vi "SimpleExportUseBookmark.vi"(4 "GraphBookmark":string, 5 "StringData":string[](array[string]), 6 "GraphReference":refnum<vi>, 7 "BookmarkTarget":string[](array[string]), 8 "error in (no error)":errorcluster, 10 "TemplateFilePath":path) -> (0 "error out":errorcluster)   [LabVIEW 2013]
uses:
  <vilib>/Utility/NIReport.llb/NI_report.lvclass
  <vilib>/Utility/NIReport.llb/Append Report Text (str wrap).vi
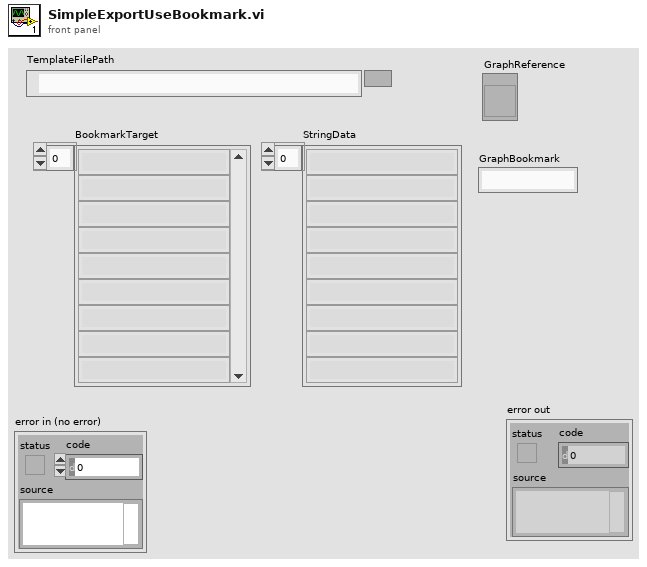
[diagram p1: front panel]
types:
  T1 = cluster{"position (excel)":cluster{"row":i32, "column":i32}, "name (excel)":string, "bookmark (word)":string}
  T2 = enum16{"Standard Report", "HTML", "Word", "Excel"}
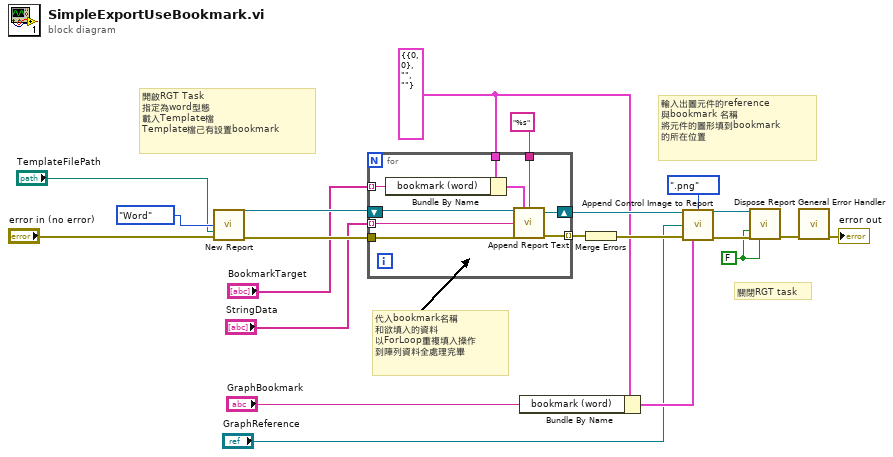
[diagram p0: block diagram]
diagram:
  w5 = FALSE ("save changes? (F)")
  w10 = T1 {"position (excel)"={"row"=0, "column"=0}, "name (excel)"="", "bookmark (word)"=""} ("MS Office parameters")
  # "關閉RGT task"
  # "輸入出圖元件的reference\n與bookmark 名稱\n將元件的圖形填到bookmark\n的所在位置"
  # "代入bookmark名稱\n和欲填入的資料\n以ForLoop重複填入操作\n到陣列資料全處理完畢"
  # "開啟RGT Task\n指定為word型態\n載入Template檔\nTemplate檔己有設置bookmark"
  n1 = call <vilib>:"New Report.vi"("report type"=T2."Word", "template (empty)"="TemplateFilePath", "error in (no error)"="error in (no error)") -> ("report out"=w19:refnum<class "NI_report.lvclass">, "error out"=w18:errorcluster)  [unwired: 11 in]
  n2 = for {
    tunnel: w10 -> [w30]
    tunnel: w18 -> [w27]
    tunnel: "BookmarkTarget" -> [w26] mode=indexing
    tunnel: "StringData" -> [w25] mode=indexing
    tunnel: "%s" ("format string (%.3f)") -> [w24]
    shift-right: [w23] -> w14
    shift-left: w19 -> [w28]
    tunnel: [w22] -> w13 mode=indexing
    n3 = Bundle By Name(cluster=w30, "bookmark (word)"=w26) -> (w29:T1)
    n4 = call-poly <vilib>:"Append Report Text.vi"("report in"=w28, "MS Office parameters"=w29, "format string (%.3f)"=w24, "text"=w25, "error in (no error)"=w27) -> ("report out"=w23:refnum<class "NI_report.lvclass">, "error out"=w22:errorcluster)  [unwired: 7 in, 2 out]
  }
  n5 = Bundle By Name(cluster=w10, "bookmark (word)"="GraphBookmark") -> (w8:T1)
  n6 = Merge Errors(w13) -> (w12:errorcluster)
  n7 = call-dynamic "Append Control Image to Report.vi"("report in"=w14, "image file type (.jpg)"=enum16{".jpg", ".png"}.".png", "ctrl reference"="GraphReference", "error in (no error)"=w12, "MS Office parameters"=w8) -> ("report out"=w7:refnum<class "NI_report.lvclass">, "error out"=w6:errorcluster)  [unwired: 7 in, 2 out]
  n8 = call-dynamic "Dispose Report.vi"("report in"=w7, "save changes? (F)"=w5, "error in (no error)"=w6, "close report? (T)"=w5) -> ("error out"=w4:errorcluster)  [unwired: 11 in]
  n9 = call <vilib>:"General Error Handler.vi"("error in (no error)"=w4) -> ("error out"=→"error out":errorcluster)  [unwired: 10 in, 4 out]
